vi "ASCII numbers to String.vi"(11 "ascii numbers":dbl[](array[numeric])) -> (3 "string":string)   [LabVIEW 2013, in "GOLPI library.lvlib"]
doc: "Converts string with real number into double format. In the case of parse error output is set to NaN."
uses:
  GOLPI library.lvlib
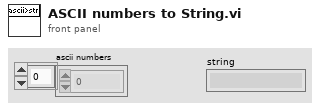
[diagram p1: front panel]
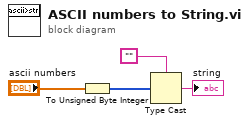
[diagram p0: block diagram]
diagram:
  n1 = To Unsigned Byte Integer(number="ascii numbers") -> (unsigned 8bit integer=w3:u8[])
  n2 = Type Cast(type="", x=w3) -> (*(type *) &x=→"string":string)
